vi "Door Locking System.vi"() -> ()   [LabVIEW 2019]
panel:
  out "String 2":string
  in  "Search Button":bool
  out "Password":string
  out "Slide":u8(slide) scale=0.0..100.0
  in  "Password":T1
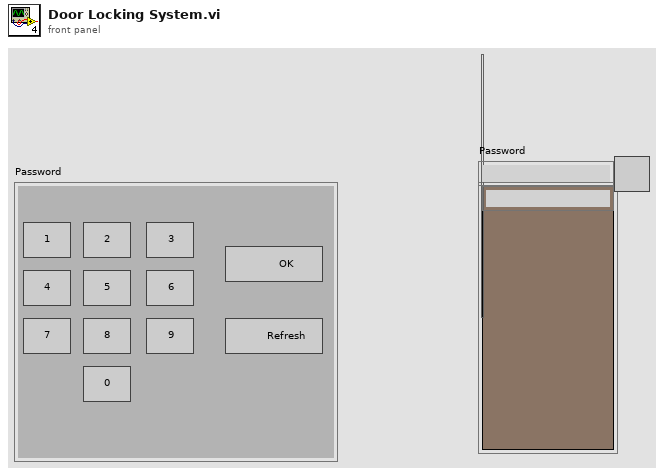
[diagram p1: front panel]
types:
  T1 = cluster{"Blank Button":bool, "Blank Button 2":bool, "Blank Button 3":bool, "Blank Button 4":bool, "Blank Button 5":bool, "Blank Button 6":bool, "Blank Button 7":bool, "Blank Button 8":bool, "Blank Button 9":bool, "Blank Button 10":bool, "OK Button":bool, "Refresh Button":bool}
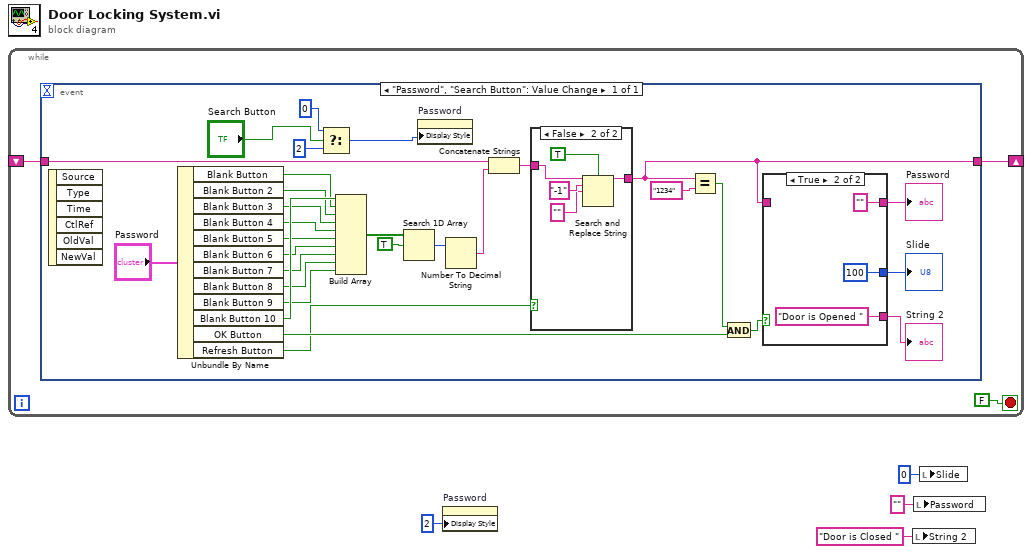
[diagram p0: block diagram]
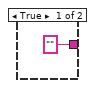
[diagram p2: hidden frame]
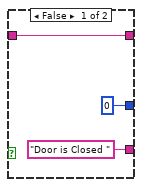
[diagram p3: hidden frame]
diagram:
  n1 = while {
    shift-right: [w6] -> _
    shift-left: _ -> [w5]
    stop <- FALSE stop-if-true
    n2 = event shown="[0] \"Password\", \"Search Button\": Value Change" {
      selector: _ -> [_]
      dyn-events: _ -> [_]
      timeout: _ -> [_]
      tunnel: [w12] -> w6
      tunnel: w5 -> [w22]
      event "Password", "Search Button": Value Change {
        n3 = event-data() -> ()  [unwired: 1 in, 6 out]
        n4 = Unbundle By Name("Password") -> ("Blank Button"=w35:bool, "Blank Button 2"=w34:bool, "Blank Button 3"=w33:bool, "Blank Button 4"=w32:bool, "Blank Button 5"=w31:bool, "Blank Button 6"=w30:bool, "Blank Button 7"=w29:bool, "Blank Button 8"=w28:bool, "Blank Button 9"=w27:bool, "Blank Button 10"=w36:bool, "OK Button"=w17:bool, "Refresh Button"=w14:bool)
        n5 = Select(t=u32 0 ("Display Style"), s="Search Button", f=u32 2 ("Display Style")) -> (s? t:f=w8:u32)
        n6 = Build Array(w36, w35, w34, w33, w32, w31, w30, w29, w28, w27) -> (w26:bool[])
        n7 = Search 1D Array(1D array=w26, element=TRUE) -> (index of element=w24:i32)  [unwired: 1 in]
        n8 = property on="Password" class="Str"("Display Style"=w8) -> ()  [unwired: 2 in, 2 out]
        n9 = Number To Decimal String(number=w24) -> (decimal integer string=w23:string)  [unwired: 1 in]
        n10 = Concatenate Strings(w22, w23) -> (w15:string)
        n11 = case shown="False" w14 {
          tunnel: w15 -> [_ w43]
          tunnel: ["" w39] -> w12
          frame True {
          }
          frame False {
            n12 = Search and Replace String(case sensitive?=TRUE ("ignore case? (F)"), input string=w43, search string="-1", replace string="" ("replace string (\"\")")) -> (result string=w39:string)  [unwired: 4 in, 3 out]
          }
        }
        n13 = Equal?(x=w12, y="1234") -> (x = y?=w18:bool)
        n14 = And(x=w18, y=w17) -> (x .and. y?=w16:bool)
        n15 = case shown="True" w16 {
          tunnel: [u8 0 ("Slide") u8 100 ("Slide")] -> w20
          tunnel: ["Door is Closed " ("String 2") "Door is Opened " ("String 2")] -> w19
          tunnel: w12 -> [w44 _]
          tunnel: [w44 "" ("Password")] -> w13
          frame False {
          }
          frame True {
          }
        }
        "Password" <- w13
        "String 2" <- w19
        "Slide" <- w20
      }
    }
  }
  n16 = property on="Password" class="Str"("Display Style"=u32 2) -> ()  [unwired: 2 in, 2 out]
  n17 = local write "String 2"("Door is Closed " ("String 2")) -> ()
  n18 = local write "Password"("" ("Password")) -> ()
  n19 = local write "Slide"(u8 0 ("Slide")) -> ()
